vi "Motors Sub 02.vi"(7 "Cluster":T1, 8 "error in":errorcluster, 11 "VISA in":refnum<visa-resource-name>) -> (0 "error out":errorcluster, 3 "VISA out":refnum<visa-resource-name>)   [LabVIEW 2010]
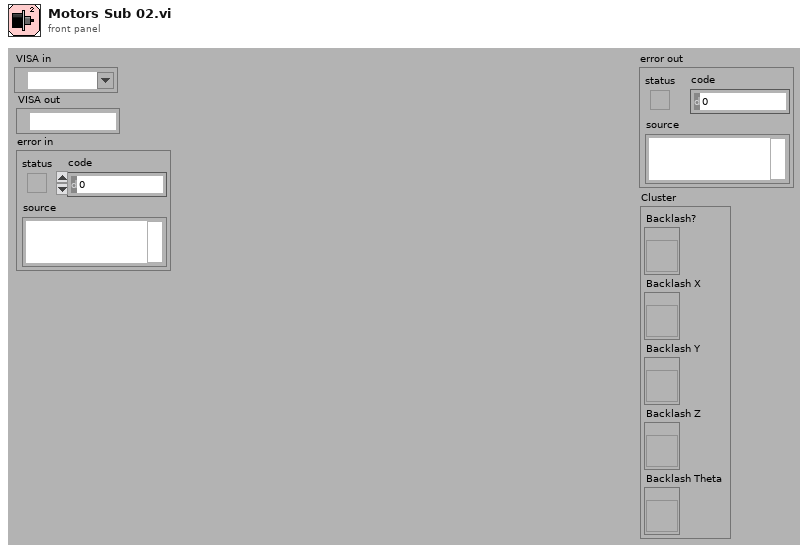
[diagram p1: front panel]
types:
  T1 = cluster{"Backlash?":refnum<vi>, "Backlash X":refnum<vi>, "Backlash Y":refnum<vi>, "Backlash Z":refnum<vi>, "Backlash Theta":refnum<vi>}
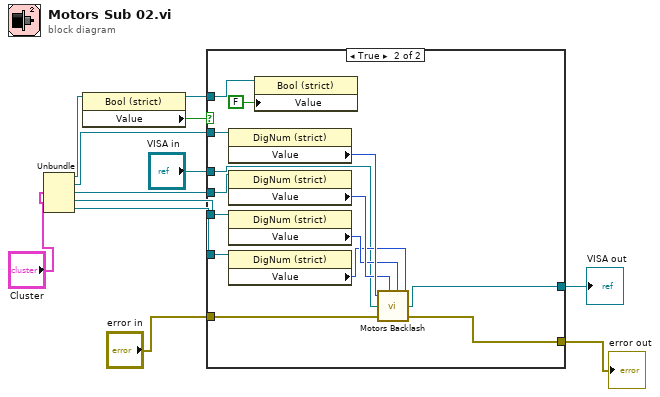
[diagram p0: block diagram]
diagram:
  n1 = Unbundle("Cluster") -> ("Backlash?"=w8:refnum<vi>, "Backlash X"=w12:refnum<vi>, "Backlash Y"=w11:refnum<vi>, "Backlash Z"=w10:refnum<vi>, "Backlash Theta"=w9:refnum<vi>)
  n2 = property on="Property Node" class="Bool (strict)"(reference=w8) -> (reference out=w6:refnum<vi>, "Value"=w7:bool)  [unwired: 1 in, 1 out]
  n3 = case shown="True" w7 {
    tunnel: [w14 w28] -> w4
    tunnel: w12 -> [_ w27]
    tunnel: w11 -> [_ w25]
    tunnel: w10 -> [_ w23]
    tunnel: w9 -> [_ w21]
    tunnel: w6 -> [_ w18]
    tunnel: "VISA in" -> [w14 w17]
    tunnel: "error in" -> [w13 w16]
    tunnel: [w13 w15] -> w2
    frame False {
    }
    frame True {
      n4 = property on="Property Node" class="DigNum (strict)"(reference=w27) -> ("Value"=w26:u32)  [unwired: 1 in, 2 out]
      n5 = property on="Property Node" class="DigNum (strict)"(reference=w25) -> ("Value"=w24:u32)  [unwired: 1 in, 2 out]
      n6 = property on="Property Node" class="DigNum (strict)"(reference=w23) -> ("Value"=w22:u32)  [unwired: 1 in, 2 out]
      n7 = property on="Property Node" class="DigNum (strict)"(reference=w21) -> ("Value"=w20:u32)  [unwired: 1 in, 2 out]
      n8 = property on="Property Node" class="Bool (strict)"(reference=w18, "Value"=FALSE) -> ()  [unwired: 1 in, 2 out]
      n9 = call "Motors Backlash.vi"("X"=w26, "Y"=w24, "VISA in"=w17, "error in"=w16, "Z"=w22, "Theta"=w20) -> ("VISA out"=w28:refnum<visa-resource-name>, "error out"=w15:errorcluster)  [unwired: 2 in]
    }
  }
  "VISA out" <- w4
  "error out" <- w2
